vi "WriteCalcDatQ.vi"(7 "DataIn":dbl[](array[numeric]), 8 "error in (no error)":errorcluster caption="entrée d'erreur (pas d'erreur)", 9 "CrvIndexIn":i32, 10 "CurCrvPointIndIn":i32, 11 "Interface en entrée":refnum<class "Interface.lvclass"> caption="DNL_LabVIEW Object in") -> (0 "error out":errorcluster caption="sortie d'erreur", 1 "CrvIndex":i32, 2 "CurCrvPointInd":i32, 3 "Interface en sortie":refnum<class "Interface.lvclass"> caption="DNL_LabVIEW Object out")   [LabVIEW 2019, in "Interface.lvclass"]
uses:
  Interface.lvclass
  Interface.lvclass/Interface.ctl
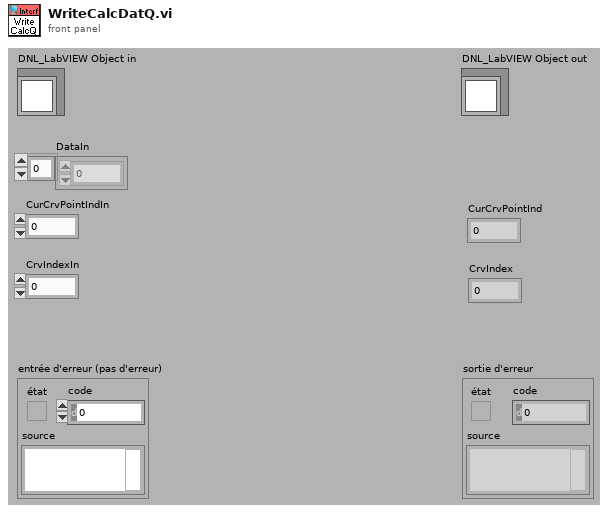
[diagram p1: front panel]
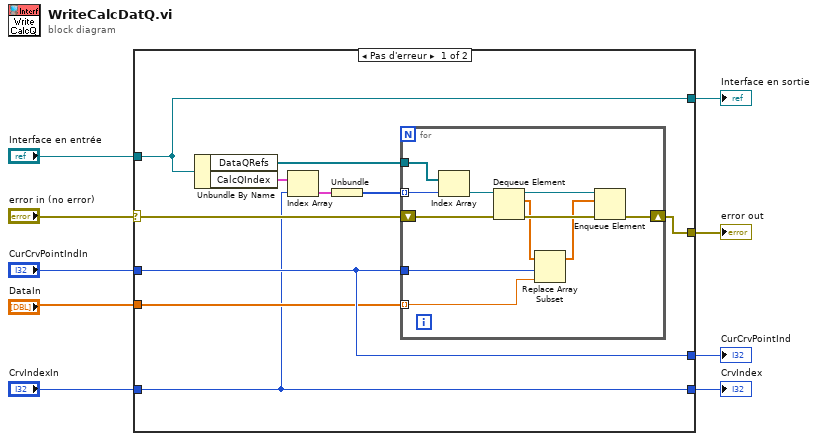
[diagram p0: block diagram]
diagram:
  n1 = case shown="Pas d'erreur" "error in (no error)" {
    selector: "error in (no error)" -> [w12 w32]
    tunnel: [w19 w32] -> w8
    tunnel: [w18 w31] -> w6
    tunnel: "Interface en entrée" -> [w18 w31]
    tunnel: "DataIn" -> [w11 _]
    tunnel: "CurCrvPointIndIn" -> [w13 _]
    tunnel: [w13 _] -> w3
    tunnel: [w10 _] -> w2
    tunnel: "CrvIndexIn" -> [w10 _]
    frame No Error {
      n2 = Unbundle By Name(w18) -> ("DataQRefs"=w17:refnum<queue>[], "CalcQIndex"=w15:cluster{"Tableau":i32[]}[])
      n3 = Index Array(array=w15, index=w10) -> (element=w16:cluster{"Tableau":i32[]})
      n4 = Unbundle(w16) -> ("Tableau"=w14:i32[])
      n5 = for {
        shift-right: [w29] -> w19
        shift-left: w12 -> [w22]
        tunnel: w11 -> [w25] mode=indexing
        tunnel: w13 -> [w24]
        tunnel: w14 -> [w20] mode=indexing
        tunnel: w17 -> [w23]
        n6 = Index Array(array=w23, index=w20) -> (element=w21:refnum<queue>)
        n7 = Dequeue Element(queue=w21, error in (no error)=w22) -> (queue out=w30:refnum<queue>, element=w27:dbl[], error out=w28:errorcluster)  [unwired: 1 in, 1 out]
        n8 = Replace Array Subset(array=w27, new element=w25, index=w24) -> (w26:dbl[])
        n9 = Enqueue Element(queue=w30, element=w26, error in (no error)=w28) -> (error out=w29:errorcluster)  [unwired: 1 in, 2 out]
      }
    }
    frame Error {
    }
  }
  "error out" <- w8
  "Interface en sortie" <- w6
  "CurCrvPointInd" <- w3
  "CrvIndex" <- w2
